vi "FPGA_DIOWriteDO_PWMDutyCycle.vi"(8 "error in (no error)":errorcluster, 9 "DO_PWM Index":i8, 10 "DO_PWMDutyCycle":u8, 11 "DIODeviceRef":T1) -> (0 "error out":errorcluster, 3 "DIODeviceRef":T1)   [LabVIEW 2017]
uses:
  <vilib>/Rock Robotics/SystemInterfaces/DIO/FPGA_DIODevRef.ctl
  <vilib>/Rock Robotics/SystemInterfaces/System/FPGA_SystemFPGA Ref Global.vi
  <vilib>/Utility/error.llb/Error Cluster From Error Code.vi
  <vilib>/rvi/errors/niLvFpgaAdjustHostInterfaceError.vi
  <vilib>/rvi/interface/nirviReadWriteControl/nirviReadWriteControl.xnode
  <vilib>/Rock Robotics/SystemInterfaces/System/FPGA_SystemFRC FPGA Ref.ctl
  <vilib>/rvi/interface/Simulation/niFpgaSimulationCallBeginRW.vi
  NiFpgaLv.dll
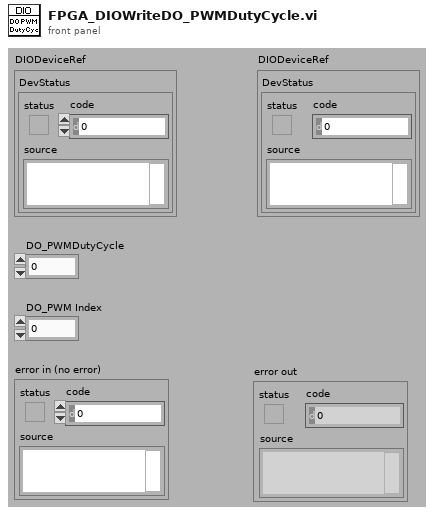
[diagram p1: front panel]
types:
  T1 = typedef "FPGA_DIODevRef.ctl" = cluster{"DevStatus":errorcluster}
  T2 = typedef "FPGA_SystemFRC FPGA Ref.ctl" = refnum<k20>
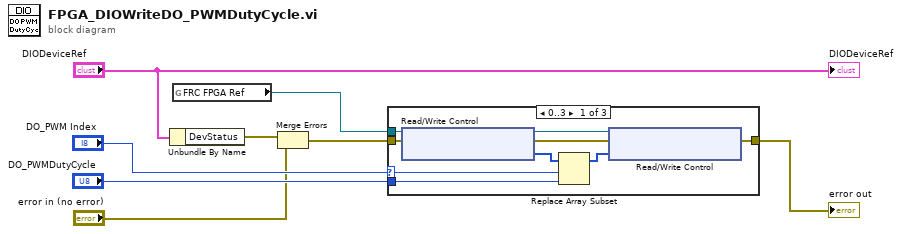
[diagram p0: block diagram]
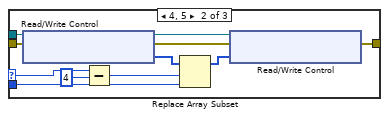
[diagram p2: hidden frame]
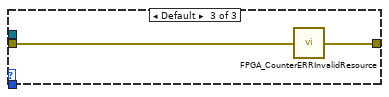
[diagram p3: hidden frame]
diagram:
  n1 = Unbundle By Name("DIODeviceRef") -> ("DevStatus"=w4:errorcluster)
  n2 = global read "FPGA_SystemFPGA Ref Global.vi" "FRC FPGA Ref"() -> (w5:T2)
  n3 = Merge Errors(w4, "error in (no error)") -> (w3:errorcluster)
  n4 = case shown="0..3" "DO_PWM Index" {
    selector: "DO_PWM Index" -> [w9 w20 _]
    tunnel: [w17 w28 w29] -> w7
    tunnel: "DO_PWMDutyCycle" -> [w12 w23 _]
    tunnel: w5 -> [w11 w22 _]
    tunnel: w3 -> [w10 w21 w30]
    frame 0..3 {
      n5 = xnode "Read/Write Control"("FPGA VI Reference In"=w11, "error in"=w10) -> ("FPGA VI Reference Out"=w16:T2, "error out"=w15:errorcluster, "DIO.PWMDutyCycleA"=w14:u8[])
      n6 = Replace Array Subset(array=w14, new element=w12, index=w9) -> (w13:u8[])
      n7 = xnode "Read/Write Control"("FPGA VI Reference In"=w16, "error in"=w15, "DIO.PWMDutyCycleA"=w13) -> ("error out"=w17:errorcluster)  [unwired: 1 out]
    }
    frame 4, 5 {
      n8 = xnode "Read/Write Control"("FPGA VI Reference In"=w22, "error in"=w21) -> ("FPGA VI Reference Out"=w27:T2, "error out"=w26:errorcluster, "DIO.PWMDutyCycleB"=w25:u8[])
      n9 = Subtract(x=w20, y=i8 4 ("x")) -> (x-y=w19:i8)
      n10 = Replace Array Subset(array=w25, new element=w23, index=w19) -> (w24:u8[])
      n11 = xnode "Read/Write Control"("FPGA VI Reference In"=w27, "error in"=w26, "DIO.PWMDutyCycleB"=w24) -> ("error out"=w28:errorcluster)  [unwired: 1 out]
    }
    frame Default {
      n12 = call <vilib>:"FPGA_CounterERRInvalidResource.vi"("error in (no error)"=w30) -> ("error out"=w29:errorcluster)
    }
  }
  "error out" <- w7
  "DIODeviceRef" <- "DIODeviceRef"
